vi "C2SD_ISM_main.vi"() -> ()   [LabVIEW 2017]
doc: "Use this template to build a user interface event handler design pattern. Use this pattern for dialog boxes and other user interfaces. You also can create and execute user-defined events that the VI can handle the same way as user interface events."
uses:
  <vilib>/Utility/error.llb/DialogType.ctl
  <vilib>/DAQmx/write.llb/DAQmx Write (Analog 1D Wfm NChan NSamp).vi
  <vilib>/DAQmx/create/channels.llb/DAQmx Create Channel (AO-Voltage-Basic).vi
  <vilib>/DAQmx/configure/timing.llb/DAQmx Timing (Sample Clock).vi
  <vilib>/DAQmx/miscellaneous.llb/DAQmx Fill In Error Info.vi
  <resource>/objmgr/daqmx.rc
panel:
  in  "Preview":enum32{"Preview"}(tab)
  in  "Y size":dbl=6.0
  in  "X Size":dbl=6.0
  out "Camera frame rate":dbl
  in  "Vertical":dbl=1024.0
  in  "Exposure time":dbl=5.0
  in  "Num of cycle":i32=2000
  out "Num of captured cycle":i32
  out "Time consumed (ms)":u32
  in  "Scan range (um)":dbl
  in  "Step size (um)":dbl=1.0
  in  "Multicolor":dbl=1.0
  in  "Z calibration 0.1/100nm":dbl
  in  "Point precision us/point":dbl=10.0
  out "Number of camera frame":dbl
  out "Acquisition rate":dbl
  out "Output Graph":waveform(dbl)[](graph)
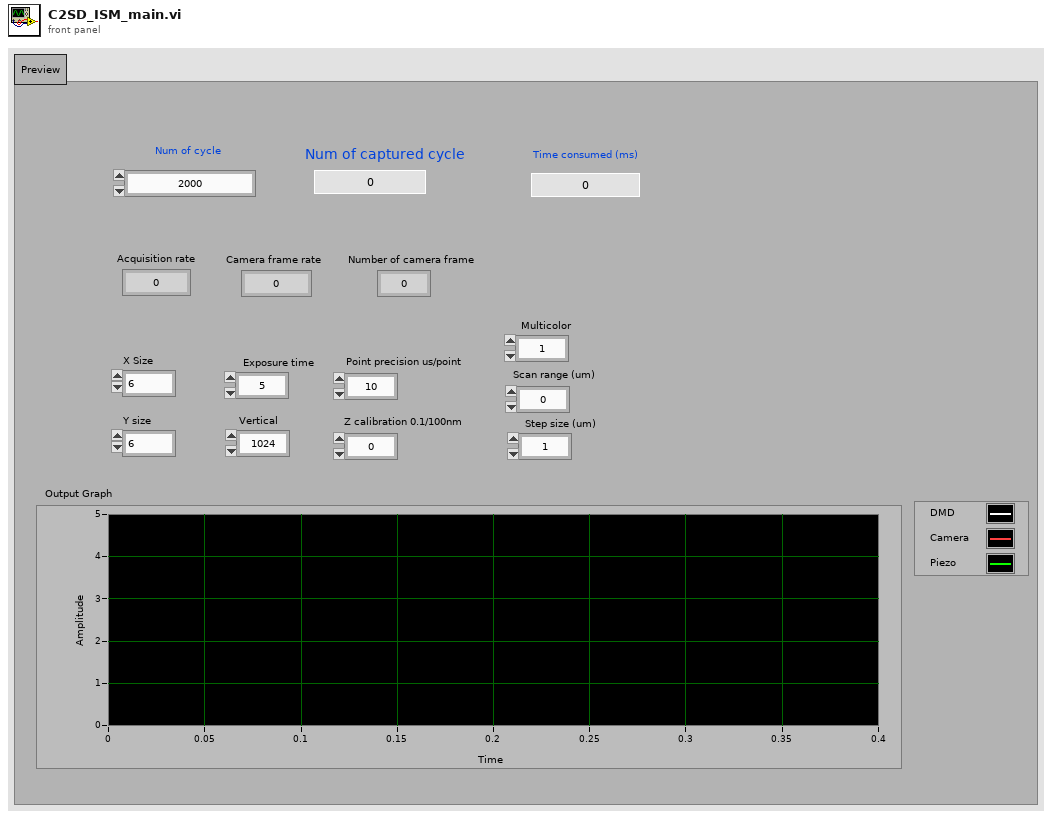
[diagram p1: front panel]
types:
  T1 = typedef "DialogType.ctl" = u16
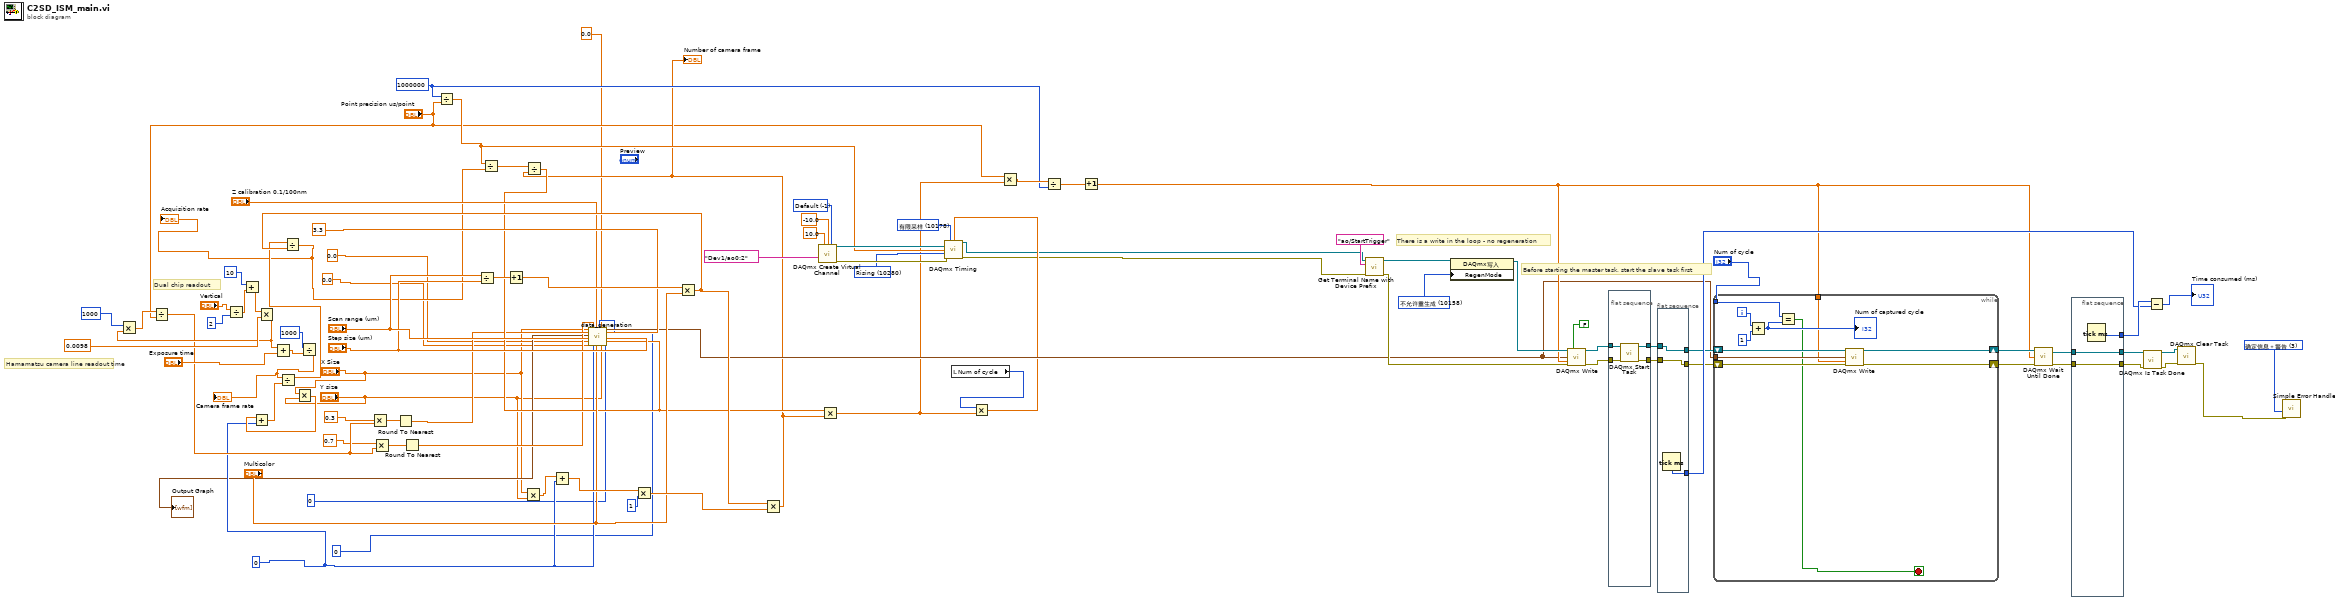
[diagram p0: block diagram]
diagram:
  w12 = 0
  w31 = 1000000
  w80 = 10158 items=["允许重生成"=10097, "不允许重生成"=10158] ("RegenMode")
  w83 = 10178 items=["有限采样"=10178, "连续采样"=10123, "硬件定时单点"=12522] ("sample mode")
  w88 = T1 3 items=["无对话框", "确定信息", "继续或停止信息", "确定信息＋警告", "继续/停止＋警告"] ("对话框类型（确定信息：1）")
  w94 = -1 items=["Default"=-1, "RSE"=10083, "Differential"=10106, "Pseudodifferential"=12529] ("output terminal configuration")
  w63 = 10280 items=["Rising"=10280, "Falling"=10171] ("active edge")
  # "Dual chip readout"
  # "Hamamatsu camera line readout time"
  # "There is a write in the loop - no regeneration"
  # "Before starting the master task, start the slave task first"
  n1 = Divide(x="Vertical", y=2) -> (x/y=w51:dbl)
  n2 = Add(x=10, y=w51) -> (x+y=w49:dbl)
  n3 = Multiply(x=w49, y=0.0098) -> (x*y=w24:dbl)
  n4 = Multiply(x=1000, y=w24) -> (x*y=w22:dbl)
  n5 = Divide(x=w22, y="Point precision us/point") -> (x/y=w20:dbl)
  n6 = Add(x=w24, y="Exposure time") -> (x+y=w53:dbl)
  n7 = Multiply(x="X Size", y="Y size") -> (x*y=w44:dbl)
  n8 = Add(x=w44, y=w12) -> (x+y=w43:dbl)
  n9 = Divide(x=1000, y=w53) -> (x/y=w48:dbl)
  "Camera frame rate" <- w48
  n10 = Divide(x=w48, y=w43) -> (x/y=w46:dbl)
  n11 = Multiply(x=0.3, y=w20) -> (x*y=w19:dbl)
  n12 = Multiply(x=0.7, y=w20) -> (x*y=w17:dbl)
  n13 = Round To Nearest(number=w19) -> (nearest integer value=w18:dbl)
  n14 = Round To Nearest(number=w17) -> (nearest integer value=w16:dbl)
  n15 = Divide(x=w31, y="Point precision us/point") -> (x/y=w33:dbl)
  n16 = Divide(x="Scan range (um)", y="Step size (um)") -> (x/y=w59:dbl)
  n17 = Increment(x=w59) -> (x+1=w58:dbl)
  n18 = Multiply(x="X Size", y="Y size") -> (x*y=w42:dbl)
  n19 = Add(x=w42, y=w12) -> (x+y=w41:dbl)
  n20 = Multiply(x=w41, y=1) -> (x*y=w57:dbl)
  n21 = Multiply(x=w58, y="Multicolor") -> (x*y=w47:dbl)
  n22 = Divide(x=w46, y=w47) -> (x/y=w9:dbl)
  "Acquisition rate" <- w9
  n23 = Divide(x=w33, y=w9) -> (x/y=w36:dbl)
  n24 = Multiply(x=w47, y=w57) -> (x*y=w27:dbl)
  "Number of camera frame" <- w27
  n25 = Divide(x=w36, y=w27) -> (x/y=w35:dbl)
  n26 = call "data_generation.vi"("X Size"="X Size", "slope"=w18, "scan range (um)"="Scan range (um)", "AmplitudeX"=0.0, "AmplitudeY"=0.0, "dwell time"=w16, "come back"=w12, "calibration"="Z calibration 0.1/100nm", "multicolor"="Multicolor", "zero point"=0, "first"=0.0, "Y size"="Y size", "AmplitudeC"=3.3, "step size (um)"="Step size (um)", "Samples per spot"=w35, "zero point 2"=0) -> ("Output Graph"=→"Output Graph":waveform(dbl)[], "XY Scan"=w29:waveform(dbl)[])  [unwired: 1 in, 1 out]
  n27 = call-poly <vilib>:"DAQmx Create Virtual Channel.vi"("maximum value"=10.0, "minimum value"=-10.0, "output terminal configuration"=w94, "physical channels"=tag "Dev1/ao0:2" ("AO channels")) -> ("task out"=w91:refnum<k21>, "error out"=w90:errorcluster)  [unwired: 10 in]
  n28 = Multiply(x=w35, y=w27) -> (x*y=w28:dbl)
  n29 = local read "Num of cycle"() -> (w62:i32)
  n30 = Multiply(x=w62, y=w28) -> (x*y=w26:dbl)
  n31 = call-poly <vilib>:"DAQmx Timing.vi"("task/channels in"=w91, "sample mode"=w83, "samples per channel"=w26, "rate"=w33, "active edge"=w63, "error in"=w90) -> ("task out"=w14:refnum<k21>, "error out"=w13:errorcluster)  [unwired: 8 in]
  n32 = Multiply(x="Point precision us/point", y=w28) -> (x*y=w32:dbl)
  n33 = Divide(x=w32, y=w31) -> (x/y=w25:dbl)
  n34 = Increment(x=w25) -> (x+1=w30:dbl)
  n35 = call "Get Terminal Name with Device Prefix.vi"("error in (no error)"=w13, "Local Terminal Name"="ao/StartTrigger" ("本地接线端名"), "task/channels in"=w14) -> ("error out"=w85:errorcluster, "task out"=w79:refnum<k21>)  [unwired: 6 in, 1 out]
  n36 = property class="DAQmx写入"(reference=w79, "RegenMode"=w80) -> (reference out=w73:refnum<k21>)  [unwired: 1 in, 1 out]
  n37 = call-poly <vilib>:"DAQmx Write.vi"("task/channels in"=w73, "auto start"=FALSE, "data"=w29, "timeout"=w30, "error in"=w85) -> ("task out"=w87:refnum<k21>, "error out"=w86:errorcluster)  [unwired: 8 in, 1 out]
  n38 = flat-sequence {
    tunnel: [w98] -> w74
    tunnel: [w97] -> w77
    tunnel: w87 -> [w96]
    tunnel: w86 -> [w95]
    frame #0 {
      n39 = call <vilib>:"DAQmx Start Task.vi"("task/channels in"=w96, "error in"=w95) -> ("task out"=w97:refnum<k21>, "error out"=w98:errorcluster)  [unwired: 12 in]
    }
  }
  n40 = flat-sequence {
    tunnel: [w101] -> w78
    tunnel: w77 -> [w100]
    tunnel: [w100] -> w76
    tunnel: [w99] -> w75
    tunnel: w74 -> [w99]
    frame #0 {
      n41 = Tick Count (ms)() -> (millisecond timer value=w101:u32)
    }
  }
  n42 = while {
    shift-right: [w108] -> w70
    shift-left: w76 -> [w109]
    shift-right: [w106] -> w69
    shift-left: w75 -> [w107]
    tunnel: "Num of cycle" -> [w110]
    tunnel: w29 -> [w104]
    tunnel: w30 -> [w103]
    i -> [w112]
    stop <- w102 stop-if-true
    n43 = Add(x=w112, y=1) -> (x+y=w105:i32)
    "Num of captured cycle" <- w105
    n44 = Equal?(x=w110, y=w105) -> (x = y?=w102:bool)
    n45 = call-poly <vilib>:"DAQmx Write.vi"("task/channels in"=w109, "data"=w104, "timeout"=w103, "error in"=w107) -> ("task out"=w108:refnum<k21>, "error out"=w106:errorcluster)  [unwired: 9 in, 1 out]
  }
  n46 = call <vilib>:"DAQmx Wait Until Done.vi"("task/channels in"=w70, "timeout (sec)"=w30, "error in"=w69) -> ("task out"=w72:refnum<k21>, "error out"=w71:errorcluster)  [unwired: 11 in]
  n47 = flat-sequence {
    tunnel: [w115] -> w82
    tunnel: w72 -> [w114]
    tunnel: [w114] -> w68
    tunnel: w71 -> [w113]
    tunnel: [w113] -> w66
    frame #0 {
      n48 = Tick Count (ms)() -> (millisecond timer value=w115:u32)
    }
  }
  n49 = call <vilib>:"DAQmx Is Task Done.vi"("task/channels in"=w68, "error in"=w66) -> ("task out"=w67:refnum<k21>, "error out"=w65:errorcluster)  [unwired: 11 in, 1 out]
  n50 = Subtract(x=w82, y=w78) -> (x-y=→"Time consumed (ms)":u32)
  n51 = call <vilib>:"DAQmx Clear Task.vi"("task in"=w67, "error in"=w65) -> ("error out"=w15:errorcluster)  [unwired: 13 in]
  n52 = call <vilib>:"Simple Error Handler.vi"("type of dialog (OK msg:1)"=w88, "error in (no error)"=w15) -> ()  [unwired: 3 in, 5 out]
